vi "Enable Input.vi"(8 "error in":errorcluster, 11 "3300 in":refnum<class "3300.lvclass">) -> (0 "error out":errorcluster, 3 "3300 out":refnum<class "3300.lvclass">)   [LabVIEW 2019, in "3300.lvlib" / "3300.lvclass"]
uses:
  Library/3300.lvclass
  C:/Users/Public/Documents/Development/builds/Instruments/Electronic Load.lvlibp/Library/Electronic Load.lvclass
  Library/3300.lvclass/3300.ctl
  Accessors/Read Local Resource.vi
  Accessors/Write Local Resource.vi
  builds/Instruments/Electronic Load.lvlibp/Accessors/Settings/Read Output Enable.vi
  <instrlib>/Agilent N330X Series/Agilent N330X Series.lvlib
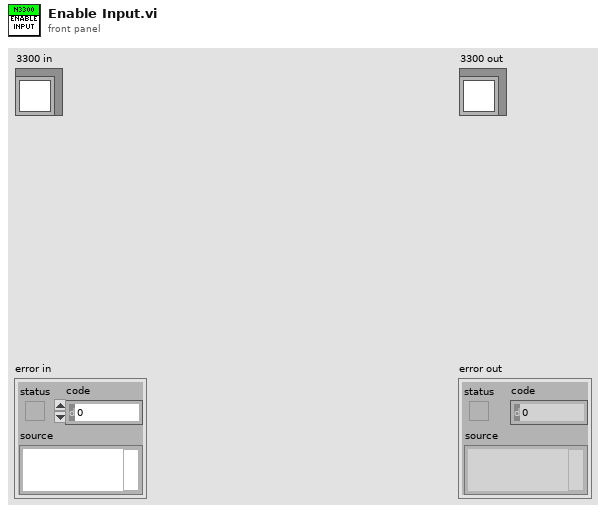
[diagram p1: front panel]
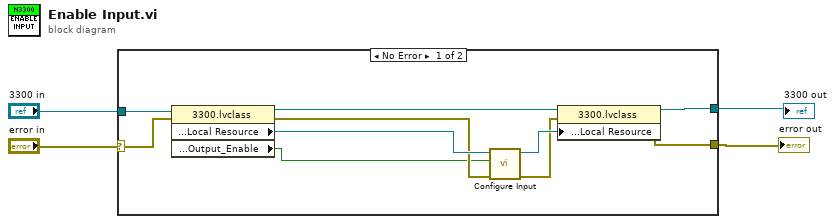
[diagram p0: block diagram]
diagram:
  n1 = case shown="No Error" "error in" {
    selector: "error in" -> [w12 w16]
    tunnel: [w11 w16] -> w1
    tunnel: [w13 w15] -> w3
    tunnel: "3300 in" -> [w10 w15]
    frame No Error {
      n2 = property class="3300.lvclass"(reference=w10, error in=w12) -> (reference out=w14:refnum<class "3300.lvclass">, error out=w6:errorcluster, "Private:Accessors:Local Resource"=w9:refnum<visa-resource-name>, "Accessors:Settings:Output_Enable"=w5:bool)
      n3 = call <instrlib>:"Configure Input.vi"("error in (no error)"=w6, "Enable Input (Enable)"=w5, "VISA resource name"=w9) -> ("error out"=w7:errorcluster, "VISA resource name out"=w8:refnum<visa-resource-name>)  [unwired: 7 in]
      n4 = property class="3300.lvclass"(reference=w14, error in=w7, "Private:Accessors:Local Resource"=w8) -> (reference out=w13:refnum<class "3300.lvclass">, error out=w11:errorcluster)
    }
    frame Error {
    }
  }
  "error out" <- w1
  "3300 out" <- w3
